vi "decimateArray.vi"(0 "Array":dbl[](array[numeric]) format="%.2f", 3 "Numeric":i32) -> (5 "Array 2":dbl[](array[numeric]) format="%.2f")   [LabVIEW 2012]
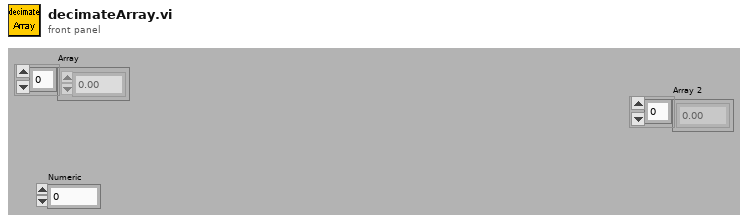
[diagram p1: front panel]
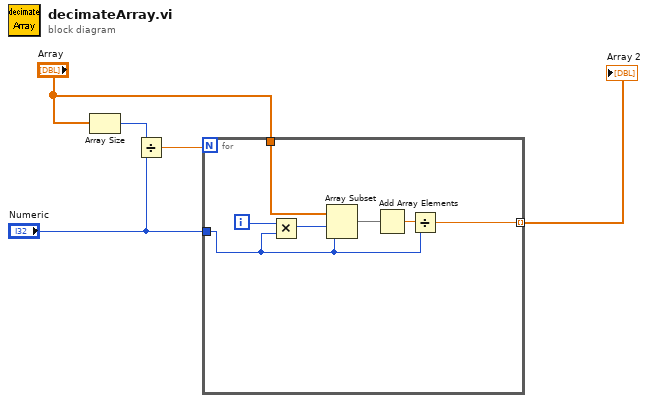
[diagram p0: block diagram]
diagram:
  n1 = Array Size(array="Array") -> (size(s)=w5:i32)
  n2 = Divide(x=w5, y="Numeric") -> (x/y=w4:dbl)
  n3 = for {
    N: w4 -> [_]
    tunnel: "Array" -> [w12]
    tunnel: "Numeric" -> [w7]
    tunnel: [w6] -> w1 mode=indexing
    i -> [w10]
    n4 = Multiply(x=w10, y=w7) -> (x*y=w11:i32)
    n5 = Array Subset(array=w12, index=w11, length=w7) -> (w9:dbl[])
    n6 = Add Array Elements(numeric array=w9) -> (sum=w8:dbl)
    n7 = Divide(x=w8, y=w7) -> (x/y=w6:dbl)
  }
  "Array 2" <- w1
